vi "locate tag.vi"(10 "tag descriptor":refnum<class "tag descriptor.lvclass">, 11 "engine configuration in":refnum<class "engine configuration.lvclass">) -> (2 "index":i32, 3 "engine configuration out":refnum<class "engine configuration.lvclass">)   [LabVIEW 2013, in "engine configuration.lvclass"]
uses:
  engine configuration.lvclass
  <vilib>/NI/Tag Bus/tag/tag descriptor.lvclass
  engine configuration.lvclass/engine configuration.ctl
  <vilib>/NI/Tag Bus/tag/tag descriptor.lvclass/tag descriptor.ctl
  <vilib>/NI/Tag Bus/tag/read tag name.vi
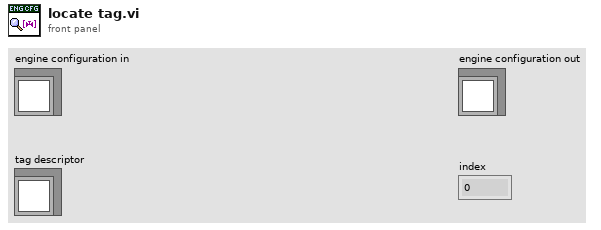
[diagram p1: front panel]
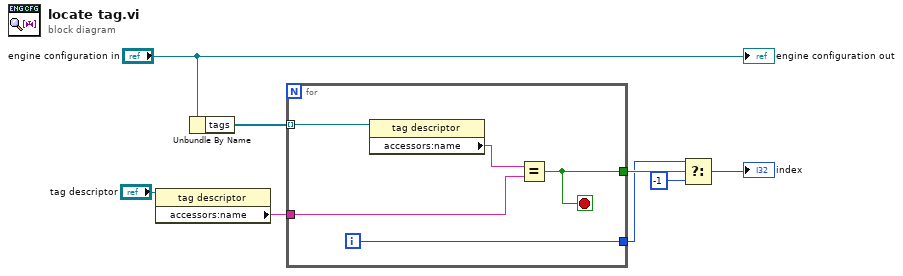
[diagram p0: block diagram]
diagram:
  n1 = property class="tag descriptor"(reference="tag descriptor") -> ("accessors:name"=w1:string)  [unwired: 1 in, 2 out]
  n2 = Unbundle By Name("engine configuration in") -> ("tags"=w7:refnum<class "tag descriptor.lvclass">[])
  n3 = for {
    tunnel: w7 -> [w10] mode=indexing
    tunnel: [w12] -> w6
    tunnel: [w11] -> w5
    tunnel: w1 -> [w9]
    i -> [w11]
    stop <- w12 stop-if-true
    n4 = property class="tag descriptor"(reference=w10) -> ("accessors:name"=w13:string)  [unwired: 1 in, 2 out]
    n5 = Equal?(x=w13, y=w9) -> (x = y?=w12:bool)
  }
  n6 = Select(t=w5, s=w6, f=-1) -> (s? t:f=→"index":i32)
  "engine configuration out" <- "engine configuration in"
